vi "Get Instrument Canonical.vi"(8 "error in (no error)":errorcluster, 11 "Driver in":refnum<class "Driver.lvclass">) -> (0 "error out":errorcluster, 2 "Canonical Name":string, 3 "Driver out":refnum<class "Driver.lvclass">)   [LabVIEW 2023, in "HAF.lvlib" / "Driver.lvclass"]
doc: "Returns the canonical name of the Instrument for this Driver that can be used to initiate a session. Must be implemented by Subclasses because there is no Visa Session available to obtain it from when it is needed. Note that this method can return an empty string IF Get Instrument Alias provides a name.\n\nThe parent implementation returns an empty string so does not need overriding where Aliases are used."
uses:
  Driver.lvclass
  Driver.lvclass/Driver.ctl
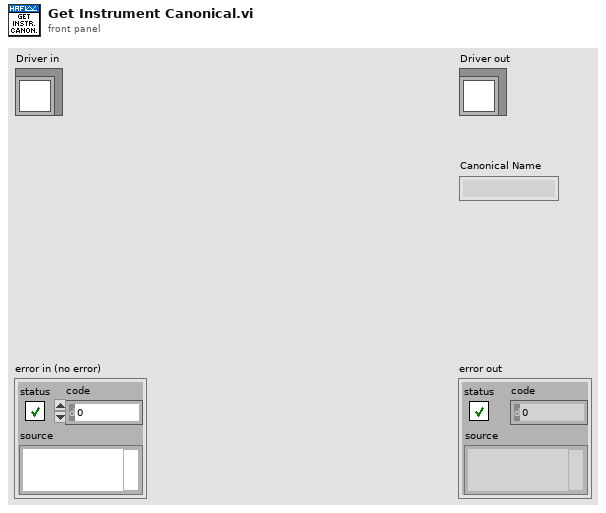
[diagram p1: front panel]
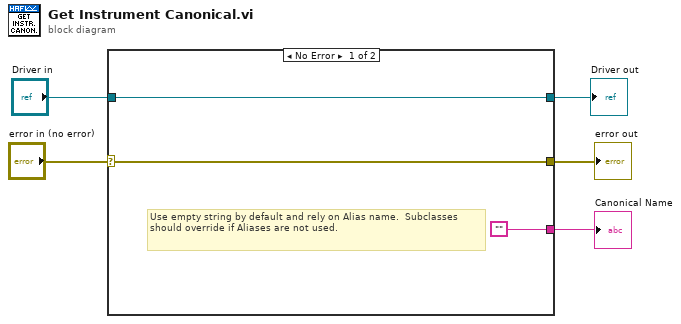
[diagram p0: block diagram]
diagram:
  n1 = case shown="No Error" "error in (no error)" {
    selector: "error in (no error)" -> [w7 w10]
    tunnel: [w7 w10] -> w2
    tunnel: [w8 w9] -> w3
    tunnel: "Driver in" -> [w8 w9]
    tunnel: ["" _] -> w1
    frame No Error {
      # "Use empty string by default and rely on Alias name.  Subclasses should override if Aliases are not used."
    }
    frame Error {
    }
  }
  "error out" <- w2
  "Driver out" <- w3
  "Canonical Name" <- w1
